vi "Build GTLT Evaluation String.vi"(8 "error in (no error)":errorcluster, 11 "Test in":refnum<class "Test.lvclass">) -> (0 "error out":errorcluster, 2 "Equals Evaluation String":string)   [LabVIEW 2018, in "Test.lvclass"]
doc: "Builds an evaluation string for a Greater Than test - can be used across different data type child classes within the test class structure."
uses:
  Test.lvclass
  566079a0-d1a1-4f45-820d-d06e3d83f950.vi
  Test Class String IDs.vi
  <vilib>/JDP Science/JSONtext/JSON text to Variant.vi
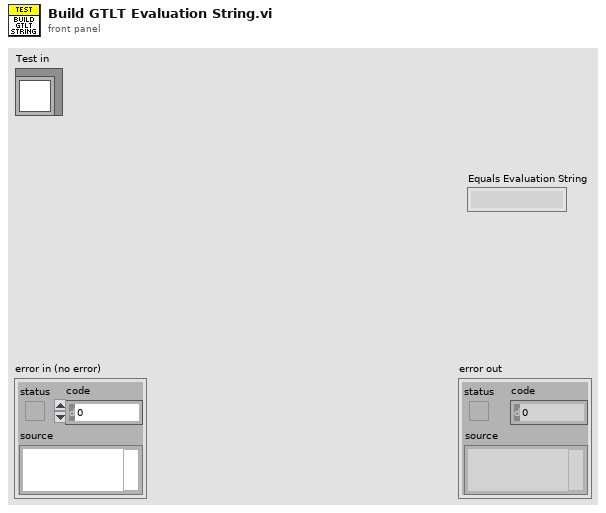
[diagram p1: front panel]
types:
  T1 = cluster{"Comparison Value 1":string, "Comparison Value 2":string, "Invert Result":string, "Assert VI Name":string, "Data Type":string, "Builder User Name":string, "Build Timestamp":string, "Failure Action":string, "Comment":string, "Assert Name":string, "Description":string, "Evaluation String":string}
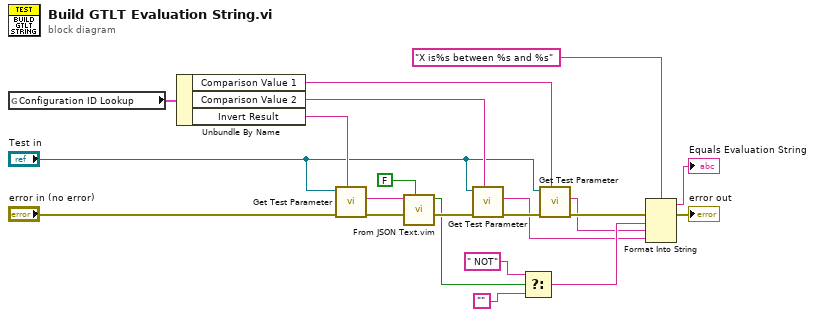
[diagram p0: block diagram]
diagram:
  n1 = global read "Test Class String IDs.vi" "Configuration ID Lookup"() -> (w17:T1)
  n2 = Unbundle By Name(w17) -> ("Comparison Value 1"=w8:string, "Comparison Value 2"=w15:string, "Invert Result"=w16:string)
  n3 = call "Get Test Parameter.vi"("Data Value ID"=w16, "error in (no error)"="error in (no error)", "Test in"="Test in") -> ("error out"=w18:errorcluster, "Test Parameter"=w13:string)  [unwired: 6 in, 1 out]
  n4 = call "From JSON Text.vim"("Data Type and Default Value"=FALSE, "error in (no error)"=w18, "JSON"=w13) -> ("error out"=w14:errorcluster, "Data out"=w6:bool)  [unwired: 7 in]
  n5 = call "Get Test Parameter.vi"("Data Value ID"=w15, "error in (no error)"=w14, "Test in"="Test in") -> ("error out"=w10:errorcluster, "Test Parameter"=w1:string)  [unwired: 6 in, 1 out]
  n6 = Select(t=" NOT" ("input 1"), s=w6, f="") -> (s? t:f=w3:string)
  n7 = call "Get Test Parameter.vi"("Data Value ID"=w8, "error in (no error)"=w10, "Test in"="Test in") -> ("error out"=w7:errorcluster, "Test Parameter"=w2:string)  [unwired: 6 in, 1 out]
  n8 = Format Into String(format string="X is%s between %s and %s", error in=w7, w3, w2, w1) -> (resulting string=→"Equals Evaluation String":string, error out=→"error out":errorcluster)  [unwired: 1 in]
